vi "Write.vi"(7 "Frame Control":T1={"final fragment (T)"=TRUE, "Frame Type (text)"=1} {"Frame Type (text)" items=["continuation"=0, "text"=1, "binary"=2, "close"=8, "ping"=9, "pong"=10]}, 8 "error in (no error)":errorcluster, 9 "Connection ID":u64, 10 "Payload":string) -> (0 "error out":errorcluster, 1 "Connection Valid":bool, 2 "bytes written":i32)   [LabVIEW 2017, in "Front Panel Publisher.lvlib" / "Websocket.lvclass"]
uses:
  Websocket.lvclass
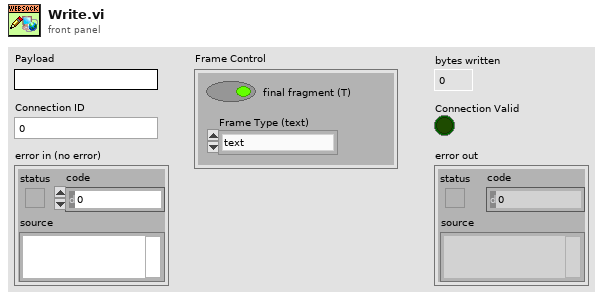
[diagram p1: front panel]
types:
  T1 = cluster{"final fragment (T)":bool, "Frame Type (text)":u8}
  T2 = typedef "FrontPanelPublisher.lvlib/Websocket.lvclass/ObjectAttributes.ctl" = cluster{"Port":u16, "TCP Refs":refnum<k5>[], "Connection IDs":u64[]}
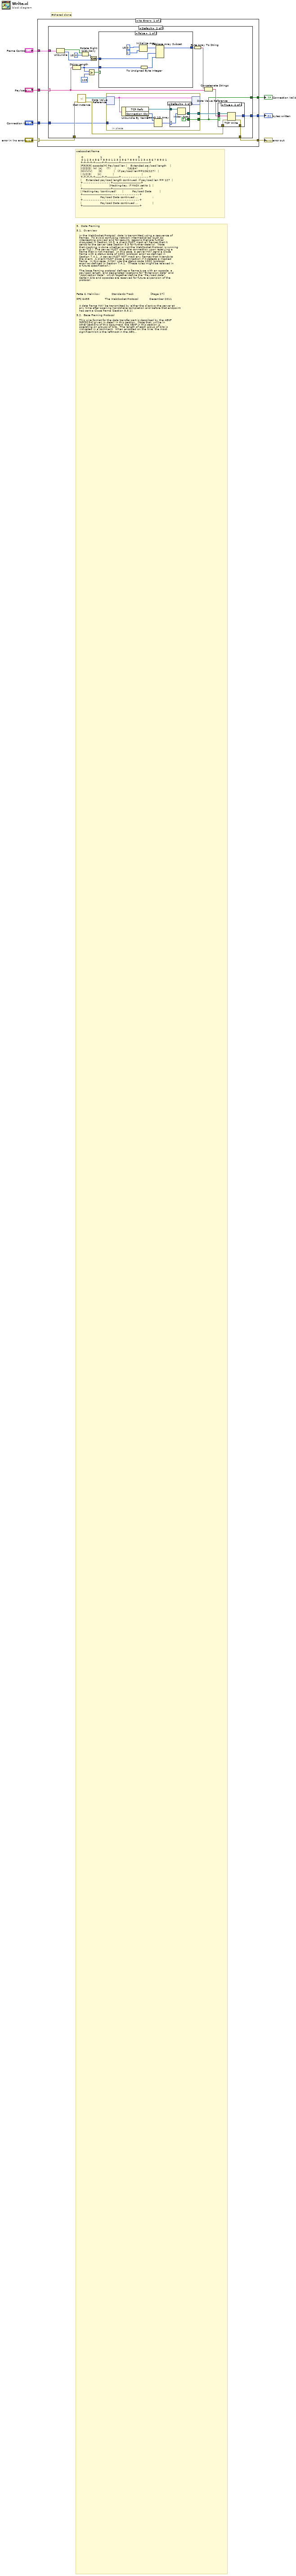
[diagram p0: block diagram]
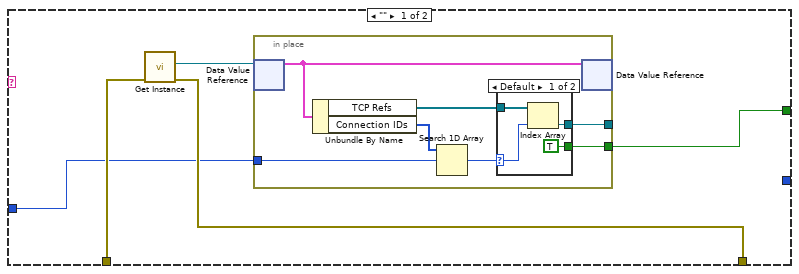
[diagram p2: hidden frame]
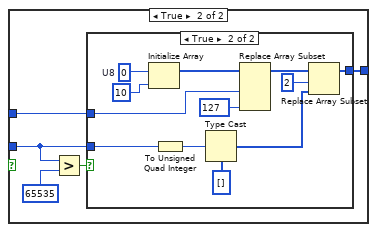
[diagram p6: hidden frame]
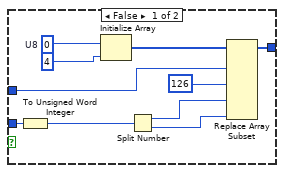
[diagram p7: hidden frame]
diagram:
  # "#shared clone"
  # "websocket frame\n \n      0                   1                   2                   3\n      0 1 2 3 4 5 6 7 8 9 0 1 2 3 4 5 6 7 8 9 0 1 2 3 4 5 6 7 8 9 0 1\n     +-+-+-+-+-------+-+-------------+-------------------------------+\n     |F|R|R|R| opcode|M| Payload len |    Extended payload length    |\n     |I|S|S|S|  (4)  |A|     (7)     |             (16/64)           |\n     |N|V|V|V|       |S|             |   (if payload len==126/127)   |\n     | |1|2|3|       |K|             |                               |\n     +-+-+-+-+-------+-+-------------+ - - - - - - - - - - - - - - - +\n     |     Extended payload length continued, if payload len == 127  |\n     + - - - - - - - - - - - - - - - +-------------------------------+\n     |                               |Masking-key, if MASK set to 1  |\n     +-------------------------------+-------------------------------+\n     | Masking-key (continued)       |          Payload Data         |\n     +-------------------------------- - - - - - - - - - - - - - - - +\n     :                     Payload Data continued ...                :\n     + - - - - - - - - - - - - - - - - - - - - - - - - - - - - - - - +\n     |                     Payload Data continued ...                |\n     +---------------------------------------------------------------+"
  # "5.  Data Framing\n\n5.1.  Overview\n\n   In the WebSocket Protocol, data is transmitted using a sequence of\n   frames.  To avoid confusing network intermediaries (such as\n   intercepting proxies) and for security reasons that are further\n   discussed in Section 10.3, a client MUST mask all frames that it\n   sends to the server (see Section 5.3 for further details).  (Note\n   that masking is done whether or not the WebSocket Protocol is running\n   over TLS.)  The server MUST close the connection upon receiving a\n   frame that is not masked.  In this case, a server MAY send a Close\n   frame with a status code of 1002 (protocol error) as defined in\n   Section 7.4.1.  A server MUST NOT mask any frames that it sends to\n   the client.  A client MUST close a connection if it detects a masked\n   frame.  In this case, it MAY use the status code 1002 (protocol\n   error) as defined in Section 7.4.1.  (These rules might be relaxed in\n   a future specification.)\n\n   The base framing protocol defines a frame type with an opcode, a\n   payload length, and designated locations for \"Extension data\" and\n   \"Application data\", which together define the \"Payload data\".\n   Certain bits and opcodes are reserved for future expansion of the\n   protocol.\n\n\n\n\n\nFette & Melnikov             Standards Track                   [Page 27]\n \nRFC 6455                 The WebSocket Protocol            December 2011\n\n\n   A data frame MAY be transmitted by either the client or the server at\n   any time after opening handshake completion and before that endpoint\n   has sent a Close frame (Section 5.5.1).\n\n5.2.  Base Framing Protocol\n\n   This wire format for the data transfer part is described by the ABNF\n   [RFC5234] given in detail in this section.  (Note that, unlike in\n   other sections of this document, the ABNF in this section is\n   operating on groups of bits.  The length of each group of bits is\n   indicated in a comment.  When encoded on the wire, the most\n   significant bit is the leftmost in the ABNF).  A high-level overview\n   of the framing is given in the following figure.  In a case of\n   conflict between the figure below and the ABNF specified later in\n   this section, the figure is authoritative.\n\n      0                   1                   2                   3\n      0 1 2 3 4 5 6 7 8 9 0 1 2 3 4 5 6 7 8 9 0 1 2 3 4 5 6 7 8 9 0 1\n     +-+-+-+-+-------+-+-------------+-------------------------------+\n     |F|R|R|R| opcode|M| Payload len |    Extended payload length    |\n     |I|S|S|S|  (4)  |A|     (7)     |             (16/64)           |\n     |N|V|V|V|       |S|             |   (if payload len==126/127)   |\n     | |1|2|3|       |K|             |                               |\n     +-+-+-+-+-------+-+-------------+ - - - - - - - - - - - - - - - +\n     |     Extended payload length continued, if payload len == 127  |\n     + - - - - - - - - - - - - - - - +-------------------------------+\n     |                               |Masking-key, if MASK set to 1  |\n     +-------------------------------+-------------------------------+\n     | Masking-key (continued)       |          Payload Data         |\n     +-------------------------------- - - - - - - - - - - - - - - - +\n     :                     Payload Data continued ...                :\n     + - - - - - - - - - - - - - - - - - - - - - - - - - - - - - - - +\n     |                     Payload Data continued ...                |\n     +---------------------------------------------------------------+\n\n   FIN:  1 bit\n\n      Indicates that this is the final fragment in a message.  The first\n      fragment MAY also be the final fragment.\n\n   RSV1, RSV2, RSV3:  1 bit each\n\n      MUST be 0 unless an extension is negotiated that defines meanings\n      for non-zero values.  If a nonzero value is received and none of\n      the negotiated extensions defines the meaning of such a nonzero\n      value, the receiving endpoint MUST _Fail the WebSocket\n      Connection_.\n\n\n\n\nFette & Melnikov             Standards Track                   [Page 28]\n \nRFC 6455                 The WebSocket Protocol            December 2011\n\n\n   Opcode:  4 bits\n\n      Defines the interpretation of the \"Payload data\".  If an unknown\n      opcode is received, the receiving endpoint MUST _Fail the\n      WebSocket Connection_.  The following values are defined.\n\n      *  %x0 denotes a continuation frame\n\n      *  %x1 denotes a text frame\n\n      *  %x2 denotes a binary frame\n\n      *  %x3-7 are reserved for further non-control frames\n\n      *  %x8 denotes a connection close\n\n      *  %x9 denotes a ping\n\n      *  %xA denotes a pong\n\n      *  %xB-F are reserved for further control frames\n\n   Mask:  1 bit\n\n      Defines whether the \"Payload data\" is masked.  If set to 1, a\n      masking key is present in masking-key, and this is used to unmask\n      the \"Payload data\" as per Section 5.3.  All frames sent from\n      client to server have this bit set to 1.\n\n   Payload length:  7 bits, 7+16 bits, or 7+64 bits\n\n      The length of the \"Payload data\", in bytes: if 0-125, that is the\n      payload length.  If 126, the following 2 bytes interpreted as a\n      16-bit unsigned integer are the payload length.  If 127, the\n      following 8 bytes interpreted as a 64-bit unsigned integer (the\n      most significant bit MUST be 0) are the payload length.  Multibyte\n      length quantities are expressed in network byte order.  Note that\n      in all cases, the minimal number of bytes MUST be used to encode\n      the length, for example, the length of a 124-byte-long string\n      can't be encoded as the sequence 126, 0, 124.  The payload length\n      is the length of the \"Extension data\" + the length of the\n      \"Application data\".  The length of the \"Extension data\" may be\n      zero, in which case the payload length is the length of the\n      \"Application data\".\n\n\n\n\n\n\n\nFette & Melnikov             Standards Track                   [Page 29]\n \nRFC 6455                 The WebSocket Protocol            December 2011\n\n\n   Masking-key:  0 or 4 bytes\n\n      All frames sent from the client to the server are masked by a\n      32-bit value that is contained within the frame.  This field is\n      present if the mask bit is set to 1 and is absent if the mask bit\n      is set to 0.  See Section 5.3 for further information on client-\n      to-server masking.\n\n   Payload data:  (x+y) bytes\n\n      The \"Payload data\" is defined as \"Extension data\" concatenated\n      with \"Application data\".\n\n   Extension data:  x bytes\n\n      The \"Extension data\" is 0 bytes unless an extension has been\n      negotiated.  Any extension MUST specify the length of the\n      \"Extension data\", or how that length may be calculated, and how\n      the extension use MUST be negotiated during the opening handshake.\n      If present, the \"Extension data\" is included in the total payload\n      length.\n\n   Application data:  y bytes\n\n      Arbitrary \"Application data\", taking up the remainder of the frame\n      after any \"Extension data\".  The length of the \"Application data\"\n      is equal to the payload length minus the length of the \"Extension\n      data\".\n\n   The base framing protocol is formally defined by the following ABNF\n   [RFC5234].  It is important to note that the representation of this\n   data is binary, not ASCII characters.  As such, a field with a length\n   of 1 bit that takes values %x0 / %x1 is represented as a single bit\n   whose value is 0 or 1, not a full byte (octet) that stands for the\n   characters \"0\" or \"1\" in the ASCII encoding.  A field with a length\n   of 4 bits with values between %x0-F again is represented by 4 bits,\n   again NOT by an ASCII character or full byte (octet) with these\n   values.  [RFC5234] does not specify a character encoding: \"Rules\n   resolve into a string of terminal values, sometimes called\n   characters.  In ABNF, a character is merely a non-negative integer.\n   In certain contexts, a specific mapping (encoding) of values into a\n   character set (such as ASCII) will be specified.\"  Here, the\n   specified encoding is a binary encoding where each terminal value is\n   encoded in the specified number of bits, which varies for each field.\n\n\n\n\n\n\n\nFette & Melnikov             Standards Track                   [Page 30]\n \nRFC 6455                 The WebSocket Protocol            December 2011\n\n\n    ws-frame                = frame-fin           ; 1 bit in length\n                              frame-rsv1          ; 1 bit in length\n                              frame-rsv2          ; 1 bit in length\n                              frame-rsv3          ; 1 bit in length\n                              frame-opcode        ; 4 bits in length\n                              frame-masked        ; 1 bit in length\n                              frame-payload-length   ; either 7, 7+16,\n                                                     ; or 7+64 bits in\n                                                     ; length\n                              [ frame-masking-key ]  ; 32 bits in length\n                              frame-payload-data     ; n*8 bits in\n                                                     ; length, where\n                                                     ; n >= 0\n\n    frame-fin               = %x0 ; more frames of this message follow\n                            / %x1 ; final frame of this message\n                                  ; 1 bit in length\n\n    frame-rsv1              = %x0 / %x1\n                              ; 1 bit in length, MUST be 0 unless\n                              ; negotiated otherwise\n\n    frame-rsv2              = %x0 / %x1\n                              ; 1 bit in length, MUST be 0 unless\n                              ; negotiated otherwise\n\n    frame-rsv3              = %x0 / %x1\n                              ; 1 bit in length, MUST be 0 unless\n                              ; negotiated otherwise\n\n    frame-opcode            = frame-opcode-non-control /\n                              frame-opcode-control /\n                              frame-opcode-cont\n\n    frame-opcode-cont       = %x0 ; frame continuation\n\n    frame-opcode-non-control= %x1 ; text frame\n                            / %x2 ; binary frame\n                            / %x3-7\n                            ; 4 bits in length,\n                            ; reserved for further non-control frames\n\n    frame-opcode-control    = %x8 ; connection close\n                            / %x9 ; ping\n                            / %xA ; pong\n                            / %xB-F ; reserved for further control\n                                    ; frames\n                                    ; 4 bits in length\n\n\n\nFette & Melnikov             Standards Track                   [Page 31]\n \nRFC 6455                 The WebSocket Protocol            December 2011\n\n\n    frame-masked            = %x0\n                            ; frame is not masked, no frame-masking-key\n                            / %x1\n                            ; frame is masked, frame-masking-key present\n                            ; 1 bit in length\n\n    frame-payload-length    = ( %x00-7D )\n                            / ( %x7E frame-payload-length-16 )\n                            / ( %x7F frame-payload-length-63 )\n                            ; 7, 7+16, or 7+64 bits in length,\n                            ; respectively\n\n    frame-payload-length-16 = %x0000-FFFF ; 16 bits in length\n\n    frame-payload-length-63 = %x0000000000000000-7FFFFFFFFFFFFFFF\n                            ; 64 bits in length\n\n    frame-masking-key       = 4( %x00-FF )\n                              ; present only if frame-masked is 1\n                              ; 32 bits in length\n\n    frame-payload-data      = (frame-masked-extension-data\n                               frame-masked-application-data)\n                            ; when frame-masked is 1\n                              / (frame-unmasked-extension-data\n                                frame-unmasked-application-data)\n                            ; when frame-masked is 0\n\n    frame-masked-extension-data     = *( %x00-FF )\n                            ; reserved for future extensibility\n                            ; n*8 bits in length, where n >= 0\n\n    frame-masked-application-data   = *( %x00-FF )\n                            ; n*8 bits in length, where n >= 0\n\n    frame-unmasked-extension-data   = *( %x00-FF )\n                            ; reserved for future extensibility\n                            ; n*8 bits in length, where n >= 0\n\n    frame-unmasked-application-data = *( %x00-FF )\n                            ; n*8 bits in length, where n >= 0\n\n5.3.  Client-to-Server Masking\n\n   A masked frame MUST have the field frame-masked set to 1, as defined\n   in Section 5.2.\n\n\n\n\n\nFette & Melnikov             Standards Track                   [Page 32]\n \nRFC 6455                 The WebSocket Protocol            December 2011\n\n\n   The masking key is contained completely within the frame, as defined\n   in Section 5.2 as frame-masking-key.  It is used to mask the \"Payload\n   data\" defined in the same section as frame-payload-data, which\n   includes \"Extension data\" and \"Application data\".\n\n   The masking key is a 32-bit value chosen at random by the client.\n   When preparing a masked frame, the client MUST pick a fresh masking\n   key from the set of allowed 32-bit values.  The masking key needs to\n   be unpredictable; thus, the masking key MUST be derived from a strong\n   source of entropy, and the masking key for a given frame MUST NOT\n   make it simple for a server/proxy to predict the masking key for a\n   subsequent frame.  The unpredictability of the masking key is\n   essential to prevent authors of malicious applications from selecting\n   the bytes that appear on the wire.  RFC 4086 [RFC4086] discusses what\n   entails a suitable source of entropy for security-sensitive\n   applications.\n\n   The masking does not affect the length of the \"Payload data\".  To\n   convert masked data into unmasked data, or vice versa, the following\n   algorithm is applied.  The same algorithm applies regardless of the\n   direction of the translation, e.g., the same steps are applied to\n   mask the data as to unmask the data.\n\n   Octet i of the transformed data (\"transformed-octet-i\") is the XOR of\n   octet i of the original data (\"original-octet-i\") with octet at index\n   i modulo 4 of the masking key (\"masking-key-octet-j\"):\n\n     j                   = i MOD 4\n     transformed-octet-i = original-octet-i XOR masking-key-octet-j\n\n   The payload length, indicated in the framing as frame-payload-length,\n   does NOT include the length of the masking key.  It is the length of\n   the \"Payload data\", e.g., the number of bytes following the masking\n   key.\n\n5.4.  Fragmentation\n\n   The primary purpose of fragmentation is to allow sending a message\n   that is of unknown size when the message is started without having to\n   buffer that message.  If messages couldn't be fragmented, then an\n   endpoint would have to buffer the entire message so its length could\n   be counted before the first byte is sent.  With fragmentation, a\n   server or intermediary may choose a reasonable size buffer and, when\n   the buffer is full, write a fragment to the network.\n\n   A secondary use-case for fragmentation is for multiplexing, where it\n   is not desirable for a large message on one logical channel to\n   monopolize the output channel, so the multiplexing needs to be free\n\n\n\nFette & Melnikov             Standards Track                   [Page 33]\n \nRFC 6455                 The WebSocket Protocol            December 2011\n\n\n   to split the message into smaller fragments to better share the\n   output channel.  (Note that the multiplexing extension is not\n   described in this document.)\n\n   Unless specified otherwise by an extension, frames have no semantic\n   meaning.  An intermediary might coalesce and/or split frames, if no\n   extensions were negotiated by the client and the server or if some\n   extensions were negotiated, but the intermediary understood all the\n   extensions negotiated and knows how to coalesce and/or split frames\n   in the presence of these extensions.  One implication of this is that\n   in absence of extensions, senders and receivers must not depend on\n   the presence of specific frame boundaries.\n\n   The following rules apply to fragmentation:\n\n   o  An unfragmented message consists of a single frame with the FIN\n      bit set (Section 5.2) and an opcode other than 0.\n\n   o  A fragmented message consists of a single frame with the FIN bit\n      clear and an opcode other than 0, followed by zero or more frames\n      with the FIN bit clear and the opcode set to 0, and terminated by\n      a single frame with the FIN bit set and an opcode of 0.  A\n      fragmented message is conceptually equivalent to a single larger\n      message whose payload is equal to the concatenation of the\n      payloads of the fragments in order; however, in the presence of\n      extensions, this may not hold true as the extension defines the\n      interpretation of the \"Extension data\" present.  For instance,\n      \"Extension data\" may only be present at the beginning of the first\n      fragment and apply to subsequent fragments, or there may be\n      \"Extension data\" present in each of the fragments that applies\n      only to that particular fragment.  In the absence of \"Extension\n      data\", the following example demonstrates how fragmentation works.\n\n      EXAMPLE: For a text message sent as three fragments, the first\n      fragment would have an opcode of 0x1 and a FIN bit clear, the\n      second fragment would have an opcode of 0x0 and a FIN bit clear,\n      and the third fragment would have an opcode of 0x0 and a FIN bit\n      that is set.\n\n   o  Control frames (see Section 5.5) MAY be injected in the middle of\n      a fragmented message.  Control frames themselves MUST NOT be\n      fragmented.\n\n   o  Message fragments MUST be delivered to the recipient in the order\n      sent by the sender.\n\n\n\n\n\n\nFette & Melnikov             Standards Track                   [Page 34]\n \nRFC 6455                 The WebSocket Protocol            December 2011\n\n\n   o  The fragments of one message MUST NOT be interleaved between the\n      fragments of another message unless an extension has been\n      negotiated that can interpret the interleaving.\n\n   o  An endpoint MUST be capable of handling control frames in the\n      middle of a fragmented message.\n\n   o  A sender MAY create fragments of any size for non-control\n      messages.\n\n   o  Clients and servers MUST support receiving both fragmented and\n      unfragmented messages.\n\n   o  As control frames cannot be fragmented, an intermediary MUST NOT\n      attempt to change the fragmentation of a control frame.\n\n   o  An intermediary MUST NOT change the fragmentation of a message if\n      any reserved bit values are used and the meaning of these values\n      is not known to the intermediary.\n\n   o  An intermediary MUST NOT change the fragmentation of any message\n      in the context of a connection where extensions have been\n      negotiated and the intermediary is not aware of the semantics of\n      the negotiated extensions.  Similarly, an intermediary that didn't\n      see the WebSocket handshake (and wasn't notified about its\n      content) that resulted in a WebSocket connection MUST NOT change\n      the fragmentation of any message of such connection.\n\n   o  As a consequence of these rules, all fragments of a message are of\n      the same type, as set by the first fragment's opcode.  Since\n      control frames cannot be fragmented, the type for all fragments in\n      a message MUST be either text, binary, or one of the reserved\n      opcodes.\n\n   NOTE: If control frames could not be interjected, the latency of a\n   ping, for example, would be very long if behind a large message.\n   Hence, the requirement of handling control frames in the middle of a\n   fragmented message.\n\n   IMPLEMENTATION NOTE: In the absence of any extension, a receiver\n   doesn't have to buffer the whole frame in order to process it.  For\n   example, if a streaming API is used, a part of a frame can be\n   delivered to the application.  However, note that this assumption\n   might not hold true for all future WebSocket extensions.\n\n\n\n\n\n\n\nFette & Melnikov             Standards Track                   [Page 35]\n \nRFC 6455                 The WebSocket Protocol            December 2011\n\n\n5.5.  Control Frames\n\n   Control frames are identified by opcodes where the most significant\n   bit of the opcode is 1.  Currently defined opcodes for control frames\n   include 0x8 (Close), 0x9 (Ping), and 0xA (Pong).  Opcodes 0xB-0xF are\n   reserved for further control frames yet to be defined.\n\n   Control frames are used to communicate state about the WebSocket.\n   Control frames can be interjected in the middle of a fragmented\n   message.\n\n   All control frames MUST have a payload length of 125 bytes or less\n   and MUST NOT be fragmented.\n\n5.5.1.  Close\n\n   The Close frame contains an opcode of 0x8.\n\n   The Close frame MAY contain a body (the \"Application data\" portion of\n   the frame) that indicates a reason for closing, such as an endpoint\n   shutting down, an endpoint having received a frame too large, or an\n   endpoint having received a frame that does not conform to the format\n   expected by the endpoint.  If there is a body, the first two bytes of\n   the body MUST be a 2-byte unsigned integer (in network byte order)\n   representing a status code with value /code/ defined in Section 7.4.\n   Following the 2-byte integer, the body MAY contain UTF-8-encoded data\n   with value /reason/, the interpretation of which is not defined by\n   this specification.  This data is not necessarily human readable but\n   may be useful for debugging or passing information relevant to the\n   script that opened the connection.  As the data is not guaranteed to\n   be human readable, clients MUST NOT show it to end users.\n\n   Close frames sent from client to server must be masked as per\n   Section 5.3.\n\n   The application MUST NOT send any more data frames after sending a\n   Close frame.\n\n   If an endpoint receives a Close frame and did not previously send a\n   Close frame, the endpoint MUST send a Close frame in response.  (When\n   sending a Close frame in response, the endpoint typically echos the\n   status code it received.)  It SHOULD do so as soon as practical.  An\n   endpoint MAY delay sending a Close frame until its current message is\n   sent (for instance, if the majority of a fragmented message is\n   already sent, an endpoint MAY send the remaining fragments before\n   sending a Close frame).  However, there is no guarantee that the\n   endpoint that has already sent a Close frame will continue to process\n   data.\n\n\n\nFette & Melnikov             Standards Track                   [Page 36]\n \nRFC 6455                 The WebSocket Protocol            December 2011\n\n\n   After both sending and receiving a Close message, an endpoint\n   considers the WebSocket connection closed and MUST close the\n   underlying TCP connection.  The server MUST close the underlying TCP\n   connection immediately; the client SHOULD wait for the server to\n   close the connection but MAY close the connection at any time after\n   sending and receiving a Close message, e.g., if it has not received a\n   TCP Close from the server in a reasonable time period.\n\n   If a client and server both send a Close message at the same time,\n   both endpoints will have sent and received a Close message and should\n   consider the WebSocket connection closed and close the underlying TCP\n   connection.\n\n5.5.2.  Ping\n\n   The Ping frame contains an opcode of 0x9.\n\n   A Ping frame MAY include \"Application data\".\n\n   Upon receipt of a Ping frame, an endpoint MUST send a Pong frame in\n   response, unless it already received a Close frame.  It SHOULD\n   respond with Pong frame as soon as is practical.  Pong frames are\n   discussed in Section 5.5.3.\n\n   An endpoint MAY send a Ping frame any time after the connection is\n   established and before the connection is closed.\n\n   NOTE: A Ping frame may serve either as a keepalive or as a means to\n   verify that the remote endpoint is still responsive.\n\n5.5.3.  Pong\n\n   The Pong frame contains an opcode of 0xA.\n\n   Section 5.5.2 details requirements that apply to both Ping and Pong\n   frames.\n\n   A Pong frame sent in response to a Ping frame must have identical\n   \"Application data\" as found in the message body of the Ping frame\n   being replied to.\n\n   If an endpoint receives a Ping frame and has not yet sent Pong\n   frame(s) in response to previous Ping frame(s), the endpoint MAY\n   elect to send a Pong frame for only the most recently processed Ping\n   frame.\n\n\n\n\n\n\nFette & Melnikov             Standards Track                   [Page 37]\n \nRFC 6455                 The WebSocket Protocol            December 2011\n\n\n   A Pong frame MAY be sent unsolicited.  This serves as a\n   unidirectional heartbeat.  A response to an unsolicited Pong frame is\n   not expected.\n\n5.6.  Data Frames\n\n   Data frames (e.g., non-control frames) are identified by opcodes\n   where the most significant bit of the opcode is 0.  Currently defined\n   opcodes for data frames include 0x1 (Text), 0x2 (Binary).  Opcodes\n   0x3-0x7 are reserved for further non-control frames yet to be\n   defined.\n\n   Data frames carry application-layer and/or extension-layer data.  The\n   opcode determines the interpretation of the data:\n\n   Text\n\n      The \"Payload data\" is text data encoded as UTF-8.  Note that a\n      particular text frame might include a partial UTF-8 sequence;\n      however, the whole message MUST contain valid UTF-8.  Invalid\n      UTF-8 in reassembled messages is handled as described in\n      Section 8.1.\n\n   Binary\n\n      The \"Payload data\" is arbitrary binary data whose interpretation\n      is solely up to the application layer.\n\n5.7.  Examples\n\n   o  A single-frame unmasked text message\n\n      *  0x81 0x05 0x48 0x65 0x6c 0x6c 0x6f (contains \"Hello\")\n\n   o  A single-frame masked text message\n\n      *  0x81 0x85 0x37 0xfa 0x21 0x3d 0x7f 0x9f 0x4d 0x51 0x58\n         (contains \"Hello\")\n\n   o  A fragmented unmasked text message\n\n      *  0x01 0x03 0x48 0x65 0x6c (contains \"Hel\")\n\n      *  0x80 0x02 0x6c 0x6f (contains \"lo\")\n\n\n\n\n\n\n\nFette & Melnikov             Standards Track                   [Page 38]\n \nRFC 6455                 The WebSocket Protocol            December 2011\n\n\n   o  Unmasked Ping request and masked Ping response\n\n      *  0x89 0x05 0x48 0x65 0x6c 0x6c 0x6f (contains a body of \"Hello\",\n         but the contents of the body are arbitrary)\n\n      *  0x8a 0x85 0x37 0xfa 0x21 0x3d 0x7f 0x9f 0x4d 0x51 0x58\n         (contains a body of \"Hello\", matching the body of the ping)\n\n   o  256 bytes binary message in a single unmasked frame\n\n      *  0x82 0x7E 0x0100 [256 bytes of binary data]\n\n   o  64KiB binary message in a single unmasked frame\n\n      *  0x82 0x7F 0x0000000000010000 [65536 bytes of binary data]\n\n5.8.  Extensibility\n\n   The protocol is designed to allow for extensions, which will add\n   capabilities to the base protocol.  The endpoints of a connection\n   MUST negotiate the use of any extensions during the opening\n   handshake.  This specification provides opcodes 0x3 through 0x7 and\n   0xB through 0xF, the \"Extension data\" field, and the frame-rsv1,\n   frame-rsv2, and frame-rsv3 bits of the frame header for use by\n   extensions.  The negotiation of extensions is discussed in further\n   detail in Section 9.1.  Below are some anticipated uses of\n   extensions.  This list is neither complete nor prescriptive.\n\n   o  \"Extension data\" may be placed in the \"Payload data\" before the\n      \"Application data\".\n\n   o  Reserved bits can be allocated for per-frame needs.\n\n   o  Reserved opcode values can be defined.\n\n   o  Reserved bits can be allocated to the opcode field if more opcode\n      values are needed.\n\n   o  A reserved bit or an \"extension\" opcode can be defined that\n      allocates additional bits out of the \"Payload data\" to define\n      larger opcodes or more per-frame bits."
  n1 = case shown="No Error" "error in (no error)" {
    selector: "error in (no error)" -> [w10 w103]
    tunnel: [w14 w103] -> w6
    tunnel: "Payload" -> [w11 _]
    tunnel: [w13 _] -> w4
    tunnel: "Frame Control" -> [w12 _]
    tunnel: "Connection ID" -> [w9 _]
    tunnel: [w8 _] -> w1
    frame No Error {
      n2 = case shown="Default" w11 {
        selector: w11 -> [_ w37]
        tunnel: [w17 w51] -> w14
        tunnel: [_ w50] -> w13
        tunnel: w12 -> [_ w45]
        tunnel: w10 -> [w18 w35]
        tunnel: w9 -> [w16 w32]
        tunnel: [w15 w31] -> w8
        frame "" {
          n3 = call "Get Instance.vi"("error in (no error)"=w18) -> ("error out"=w17:errorcluster, "DVRRefOut"=w19:refnum<data-value>)  [unwired: 6 in, 3 out]
          n4 = in-place {
            in-place-border: [w20] -> _
            in-place-border: w16 -> [w24]
            in-place-border: [w22] -> w15
            n5 = in-place-dvr #1(w19) -> (w26:T2)  [unwired: 1 out]
            n6 = Unbundle By Name(w26) -> ("TCP Refs"=w21:refnum<k5>[], "Connection IDs"=w25:u64[])
            n7 = Search 1D Array(1D array=w25, element=w24) -> (index of element=w23:i32)  [unwired: 1 in]
            n8 = case shown="Default" w23 {
              selector: w23 -> [w29 _]
              tunnel: [TRUE _] -> w22
              tunnel: w21 -> [w28 _]
              tunnel: [w27 _] -> w20
              frame Default {
                n9 = Index Array(array=w28, index=w29) -> (element=w27:refnum<k5>)
              }
              frame -1 {
              }
            }
            n10 = in-place-dvr #1(w26) -> ()  [unwired: 2 out]
          }
        }
        frame Default {
          w47 = u8 0  # U8
          n11 = Unbundle(w45) -> ("final fragment (T)"=w46:bool, "Frame Type (text)"=w49:u8)
          n12 = String Length(string=w37) -> (length=w39:i32)
          n13 = call "Get Instance.vi"("error in (no error)"=w35) -> ("error out"=w33:errorcluster, "DVRRefOut"=w36:refnum<data-value>)  [unwired: 6 in, 3 out]
          n14 = Rotate Right With Carry(2:w47, 3:w46) -> (0:w48:u8)  [unwired: 1 out]
          n15 = Greater?(x=w39, y=125 ("upper limit")) -> (0:w43:bool)
          n16 = Or(x=w48, y=w49) -> (x .or. y?=w38:u8)
          n17 = case shown="False" w43 {
            tunnel: w39 -> [w75 w77]
            tunnel: [w74 w78] -> w40
            tunnel: w38 -> [w69 w76]
            frame False {
              w72 = u8 0  # U8
              n18 = Initialize Array(w72, 2 ("dimension size")) -> (w71:u8[])
              n19 = To Unsigned Byte Integer(number=w75) -> (unsigned 8bit integer=w70:u8)
              n20 = Replace Array Subset(array=w71, new element #1=w69, new element #2=w70) -> (w74:u8[])  [unwired: 2 in]
            }
            frame True {
              n21 = Greater?(x=w77, y=65535) -> (0:w79:bool)
              n22 = case shown="True" w79 {
                tunnel: w77 -> [w90 w102]
                tunnel: [w88 w100] -> w78
                tunnel: w76 -> [w84 w92]
                frame False {
                  w86 = u8 0  # U8
                  n23 = To Unsigned Word Integer(number=w90) -> (unsigned 16bit integer=w89:u16)
                  n24 = Initialize Array(w86, 4 ("dimension size")) -> (w85:u8[])
                  n25 = Split Number(x=w89) -> (hi(x)=w82:u8, lo(x)=w81:u8)
                  n26 = Replace Array Subset(array=w85, new element #1=w84, new element #2=u8 126 ("U8"), new element #3=w82, new element #4=w81) -> (w88:u8[])  [unwired: 4 in]
                }
                frame True {
                  w95 = u8 0  # U8
                  n27 = Initialize Array(w95, 10 ("dimension size")) -> (w94:u8[])
                  n28 = To Unsigned Quad Integer(1:w102) -> (0:w99:u64)
                  n29 = Type Cast(type=u8[] [], x=w99) -> (*(type *) &x=w91:u8[])
                  n30 = Replace Array Subset(array=w94, new element #1=w92, new element #2=u8 127 ("U8")) -> (w101:u8[])  [unwired: 2 in]
                  n31 = Replace Array Subset(array=w101, new element=w91, index=2) -> (w100:u8[])
                }
              }
            }
          }
          n32 = in-place {
            in-place-border: [w58] -> w34
            in-place-border: w32 -> [w62]
            in-place-border: [w60] -> w31
            n33 = in-place-dvr #2(w36) -> (w64:T2)  [unwired: 1 out]
            n34 = Unbundle By Name(w64) -> ("TCP Refs"=w59:refnum<k5>[], "Connection IDs"=w63:u64[])
            n35 = Search 1D Array(1D array=w63, element=w62) -> (index of element=w61:i32)  [unwired: 1 in]
            n36 = case shown="Default" w61 {
              selector: w61 -> [w67 _]
              tunnel: [TRUE _] -> w60
              tunnel: w59 -> [w66 _]
              tunnel: [w65 _] -> w58
              frame Default {
                n37 = Index Array(array=w66, index=w67) -> (element=w65:refnum<k5>)
              }
              frame -1 {
              }
            }
            n38 = in-place-dvr #2(w64) -> ()  [unwired: 2 out]
          }
          n39 = Byte Array To String(unsigned byte array=w40) -> (string=w41:string)
          n40 = Concatenate Strings(w41, w37) -> (w42:string)
          n41 = case shown="True" w31 {
            tunnel: [w52 w57] -> w51
            tunnel: [_ w56] -> w50
            tunnel: w42 -> [_ w55]
            tunnel: w34 -> [_ w54]
            tunnel: w33 -> [w52 w53]
            frame False {
            }
            frame True {
              n42 = TCP Write(connection ID=w54, data in=w55, error in (no error)=w53) -> (bytes written=w56:i32, error out=w57:errorcluster)  [unwired: 1 in, 1 out]
            }
          }
        }
      }
    }
    frame Error {
    }
  }
  "error out" <- w6
  "bytes written" <- w4
  "Connection Valid" <- w1
